vi "Read RP Instrument.vi"(8 "error in (no error)":errorcluster, 11 "Red Pitaya Lock-in Driver in":refnum<class "Red Pitaya Lock-in Driver.lvclass">) -> (0 "error out":errorcluster, 2 "RP Instrument.lvclass":refnum<class "RP Instrument.lvclass">, 3 "Red Pitaya Lock-in Driver out":refnum<class "Red Pitaya Lock-in Driver.lvclass">)   [LabVIEW 2019, in "Red Pitaya Lock-in Driver.lvclass"]
uses:
  Red Pitaya Lock-in Driver.lvclass
  RP Instrument/RP Instrument.lvclass
  Red Pitaya Lock-in Driver.lvclass/Red Pitaya Lock-in Driver.ctl
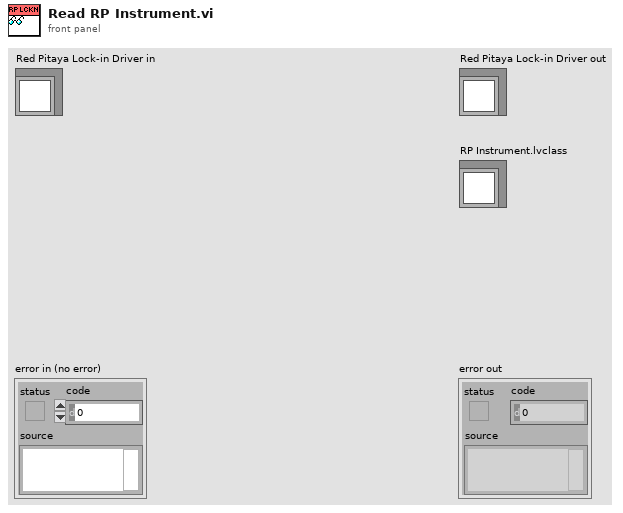
[diagram p1: front panel]
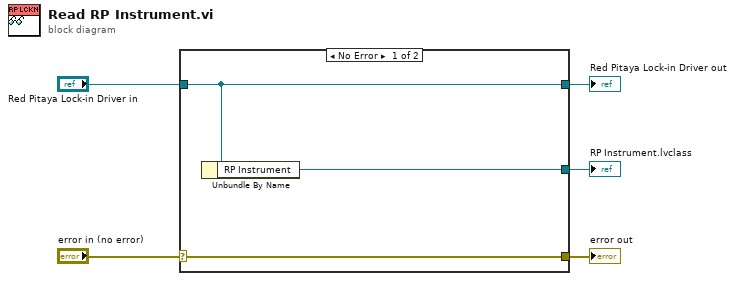
[diagram p0: block diagram]
diagram:
  n1 = case shown="No Error" "error in (no error)" {
    selector: "error in (no error)" -> [w8 w9]
    tunnel: [w8 w9] -> w4
    tunnel: [w7 w10] -> w2
    tunnel: "Red Pitaya Lock-in Driver in" -> [w7 w10]
    tunnel: [w6 _] -> w1
    frame No Error {
      n2 = Unbundle By Name(w7) -> ("RP Instrument"=w6:refnum<class "RP Instrument.lvclass">)
    }
    frame Error {
    }
  }
  "error out" <- w4
  "Red Pitaya Lock-in Driver out" <- w2
  "RP Instrument.lvclass" <- w1
